vi "Set Number Of Tests [NUM].vi"(7 "Micropulse # In":i32, 8 "error in (no error)":errorcluster) -> (0 "error out":errorcluster, 2 "Test No. Added":u32, 5 "Micropulse # Out":i32)   [LabVIEW 2026, in "MicroPulse_Driver.lvlib"]
doc: "This command specifies the number of conventional tests through which MicroPulse multiplexes when in the CAL 0, STP 0, STR 0 and fly modes.\nIn addition, the NUM command specifies the number of conventional tests to which commands using 0 test number apply.\nParameters:\n<No.> : Number of tests used. 1 to 255\n\nExample:\nNUM 50\nSets a test sequence from 1 to 50\nAll enabled tests from 1 to 50 will be performed.\n\nNUM 10\nGAN 0 40\nTests 1 to 10 gain 10dB.\n\nNUM 5\nGAN 0 80\nTests 1 to 5 gain 20dB."
uses:
  MicroPulse_Driver.lvlib
  Private/MP-Registry Action-Enum.ctl
panel:
  in  "Test Group?":bool caption="Test Group? [def: F]"
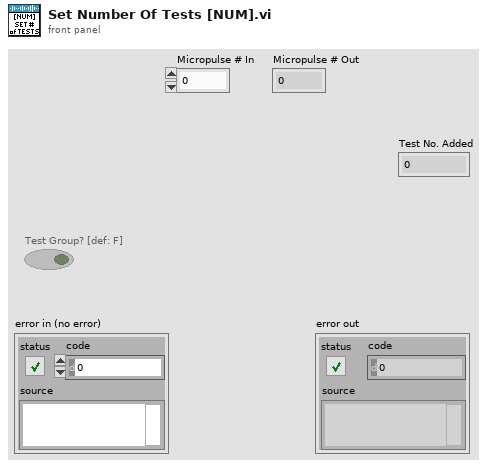
[diagram p1: front panel]
types:
  T1 = typedef "MicroPulse_Driver.lvlib/MP-Registry Action-Enum.ctl" = enum16{"Read", "Add Test", "Add Command", "Add Gate Command", "Add Encoder Command", "Clear Command  List", "Set Registry", "Set System Details", "Set DOF", "Set Velocity", "Disable Asynch Reads", "Enable Asynch Reads", "Add Connection", "Disconnect", "Shutdown"}
  T2 = typedef "MicroPulse_Driver.lvlib/MP-Registry Data-Cluster.ctl" = cluster{"Instrument Type":T3, "Serial #":u64, "Sample Frequency":T4, "dt (us)":dbl, "DOF":T5, "Material Velocity":dbl, "Asynch Reads":T6, "NUM of Tests":u32, "System Details":T7, "Gates":T9[], "Encoders":T16[], "CMD LUT":variant, "Command List":string}
  T3 = typedef "MicroPulse_Driver.lvlib/MP - instrument type.ctl" = enum16{"MicroPulse 5", "LT1", "LT2", "LTPA", "MPLT", "MicroPulse 6", "PipeScanner", "<MicroPulse>", "Micropulse 4", "Simulated Data"}
  T4 = typedef "MicroPulse_Driver.lvlib/MP - sample frequency.ctl" = enum16{"Use Default", "200MHz (LT2 only)", "100MHz", "50MHz", "25MHz", "10MHz"}
  T5 = typedef "MicroPulse_Driver.lvlib/MP - data output format.ctl" = enum16{"", "8-bit Mode", "10-bit Mode", "12-bit Mode", "16-bit Mode", "8-bit Log Mode", "12-bit Packed Mode"}
  T6 = typedef "MicroPulse_Driver.lvlib/MP - asynch read mode.ctl" = enum16{"Disabled", "Enabled"}
  T7 = typedef "MicroPulse_Driver.lvlib/MP - general system status.ctl" = cluster{"System Type":T3, "Serial No.":u64, "Channels":cluster{"Conv":u8, "PA":u16, "Extra":u32}, "Sample Frequency":cluster{"Default":u8, "Actual":u8}, "Software Versions":string, "Data Output Format":cluster{"Default":T5, "Actual":T5}, "Temperatures":cluster{"System":u8, "Processor":u8, "Slave Sys":u8, "Slave Proc":u8}, "Tx Buffer Size":u32, "System Error":string, "No. of Cards":u8, "DAC Gain":i16, "Uptimes":cluster{"since Power":u32, "since RSTS":u32, "since SRST":u32}, "Voltages":cluster{"Nominal":dbl, "Measured":dbl, "Difference":dbl}[], "Interface Cards":T8[]}
  T8 = typedef "MicroPulse_Driver.lvlib/MP - interface card status.ctl" = cluster{"Status":u8, "Map":u8, "Board - T":u8, "FPGA - T":u8, "PAIF Status":string, "Version":string}
  T9 = typedef "MicroPulse_Driver.lvlib/MP - Registry Gates.ctl" = cluster{"Display Gate":T10, "ETM Mode":T11, "Echo Gate":T12, "Insp Gates":T13[]}
  T10 = typedef "MicroPulse_Driver.lvlib/MP - display gate.ctl" = cluster{"Start":dbl, "Length":dbl}
  T11 = typedef "MicroPulse_Driver.lvlib/MP - echo gate mode.ctl" = enum16{"Echo Trigger OFF", "Echo Gate Display Mode", "Echo Trigger ON", "Multi Gate or FMC Mode", "Reserved", "PA - Echo Trigger ON"}
  T12 = typedef "MicroPulse_Driver.lvlib/MP - echo gate parameters.ctl" = cluster{"Start (us)":dbl, "Length (us)":dbl, "Threshold":u16, "Colour":u32}
  T13 = typedef "MicroPulse_Driver.lvlib/MP - multigate inspection gate parameters.ctl" = cluster{"Start (us)":dbl, "Length (us)":dbl, "Threshold":u16, "Enabled?":bool, "Max # Peaks":u16, "Hysteresis":T14, "Mode":T15, "Inverted?":bool, "Colour ":u32}
  T14 = typedef "MicroPulse_Driver.lvlib/MP - hysteresis level.ctl" = enum16{"None", "3dB", "6dB", "9dB", "12dB"}
  T15 = typedef "MicroPulse_Driver.lvlib/MP - multigate mode.ctl" = enum16{"1st Peak in Gate", "Largest Peak In Gate", "All Peaks In Gate", "1st Threshold Crossing"}
  T16 = typedef "MicroPulse_Driver.lvlib/MP - encoder settings.ctl" = cluster{"Encoder Type":T17, "Counts/mm":u32, "Enable Termination?":bool, "Multiplier":u32, "Backlash Period (s)":dbl, "Encoder Filter":u32}
  T17 = typedef "MicroPulse_Driver.lvlib/MP - encoder type.ctl" = enum16{"Quadrature", "Step/Direction"}
  T18 = typedef "MicroPulse_Driver.lvlib/TCP config.ctl" = cluster{"Connection ID":refnum<k5>, "IP address":string, "host port":u16, "OC timeout":i32, "Read timeout":i32, "Write timeout":i32}
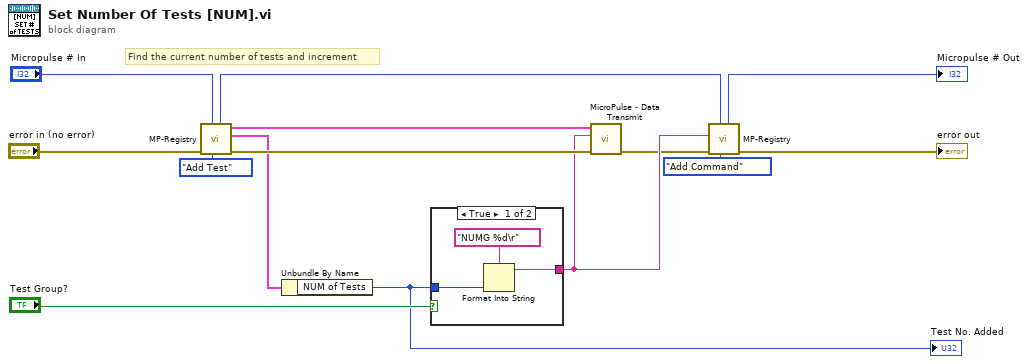
[diagram p0: block diagram]
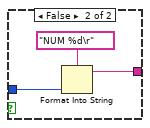
[diagram p2: hidden frame]
diagram:
  # "Find the current number of tests and increment"
  n1 = call "MP-Registry.vi"("Action"=MP-Registry_Action-Enum."Add Test", "Micropulse # In"="Micropulse # In", "error in (no error)"="error in (no error)") -> ("error out"=w12:errorcluster, "Micropulse Data"=w2:T2, "TCP config"=w11:T18, "Micropulse # Out"=w7:i32)  [unwired: 5 in]
  n2 = Unbundle By Name(w2) -> ("NUM of Tests"=w1:u32)
  "Test No. Added" <- w1
  n3 = case shown="True" "Test Group?" {
    tunnel: w1 -> [w16 w19]
    tunnel: [w15 w18] -> w10
    frame True {
      n4 = Format Into String(format string="NUMG %d\r", w16) -> (resulting string=w15:string)  [unwired: 2 in, 1 out]
    }
    frame False {
      n5 = Format Into String(format string="NUM %d\r", w19) -> (resulting string=w18:string)  [unwired: 2 in, 1 out]
    }
  }
  n6 = call "MicroPulse - Data Transmit.vi"("error in (no error)"=w12, "data"=w10, "TCP config"=w11) -> ("error out"=w8:errorcluster)  [unwired: 6 in, 2 out]
  n7 = call "MP-Registry.vi"("Action"=MP-Registry_Action-Enum."Add Command", "Micropulse # In"=w7, "error in (no error)"=w8, "Data in"=w10) -> ("error out"=→"error out":errorcluster, "Micropulse # Out"=→"Micropulse # Out":i32)  [unwired: 4 in, 2 out]
